vi "MotorOnOff.vi"(7 "#Axis":i32, 8 "error in":errorcluster, 10 "Enabled":bool, 11 "VISA resource":refnum<visa-resource-name>) -> (0 "error out":errorcluster)   [LabVIEW 2012, in "ESP300.lvlib"]
uses:
  <instrlib>/ESP300/ESP300.lvlib
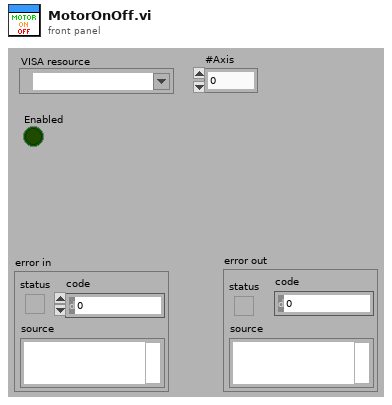
[diagram p1: front panel]
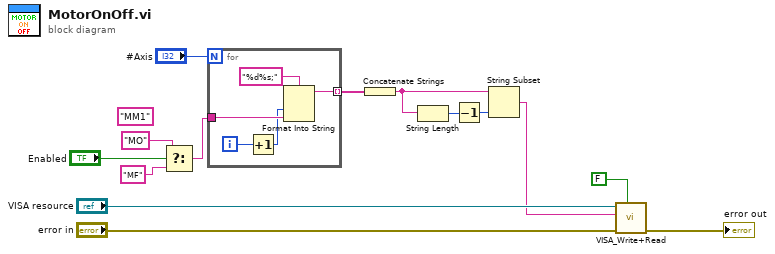
[diagram p0: block diagram]
diagram:
  (unwired) "MM1"
  n1 = Select(t="MO" ("format string"), s="Enabled", f="MF" ("format string")) -> (s? t:f=w2:string)
  n2 = for {
    N: "#Axis" -> [_]
    tunnel: [w18] -> w11 mode=indexing
    tunnel: w2 -> [w17]
    i -> [w16]
    n3 = Increment(x=w16) -> (x+1=w15:i32)
    n4 = Format Into String(format string="%d%s;", w15, w17) -> (resulting string=w18:string)  [unwired: 2 in, 1 out]
  }
  n5 = Concatenate Strings(w11) -> (w5:string)
  n6 = String Length(string=w5) -> (length=w7:i32)
  n7 = Decrement(x=w7) -> (x-1=w6:i32)
  n8 = String Subset(string=w5, length (rest)=w6) -> (substring=w4:string)  [unwired: 1 in]
  n9 = call <instrlib>:"VISA_Write+Read.vi"("Read?"=FALSE, "error in (no error)"="error in", "Write Buffer"=w4, "VISA resource name"="VISA resource") -> ("error out"=→"error out":errorcluster)  [unwired: 5 in, 2 out]
